vi "Read Latest Frame.vi"(8 "error in (no error)":errorcluster, 9 "Read Timeout (ms)":i32=100, 11 "MJPEG Reader in":refnum<data-value>) -> (0 "error out":errorcluster, 2 "Frame":string, 3 "MJPEG Reader out":refnum<data-value>)   [LabVIEW 2015, in "MJPEG Reader.lvclass"]
uses:
  MJPEG Reader.lvclass
  Get Image State.ctl
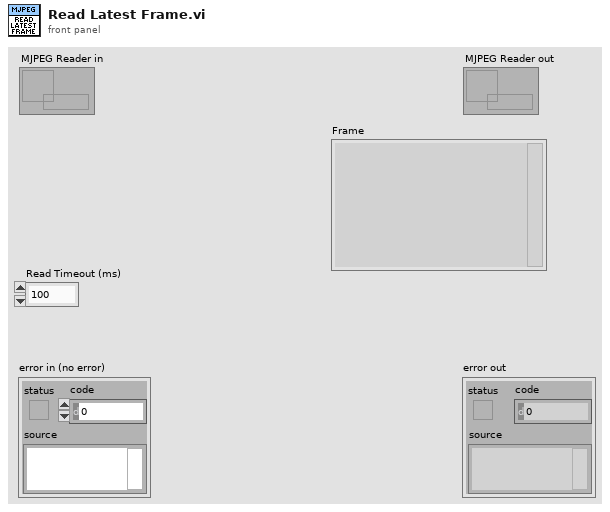
[diagram p1: front panel]
types:
  T1 = typedef "MJPEG Reader.lvclass/Get Image State.ctl" = enum16{"Read First Frame", "Check Most Recent", "Check Image"}
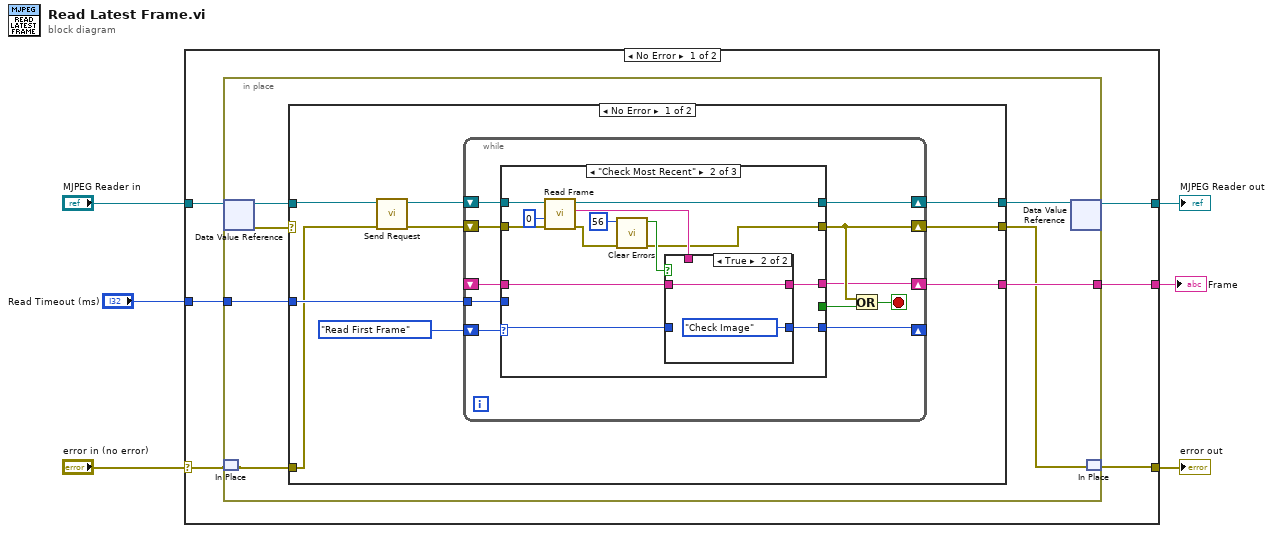
[diagram p0: block diagram]
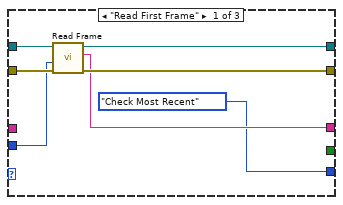
[diagram p2: hidden frame]
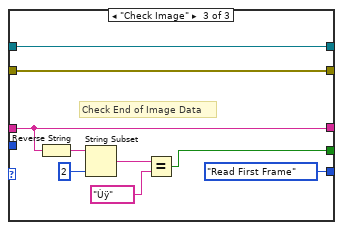
[diagram p4: hidden frame]
diagram:
  n1 = case shown="No Error" "error in (no error)" {
    selector: "error in (no error)" -> [w11 w76]
    tunnel: [w10 w76] -> w5
    tunnel: [w9 w75] -> w3
    tunnel: "MJPEG Reader in" -> [w12 w75]
    tunnel: "Read Timeout (ms)" -> [w8 _]
    tunnel: [w7 _] -> w1
    frame No Error {
      n2 = in-place {
        in-place-border: w8 -> [w15]
        in-place-border: [w14] -> w7
        n3 = in-place-dvr #1(w12) -> (w18:refnum<class "MJPEG Reader.lvclass">, w19:errorcluster)
        n4 = in-place-match #2(w11) -> (w16:errorcluster)
        n5 = case shown="No Error" w19 {
          selector: w19 -> [_ w73]
          tunnel: w18 -> [w23 w74]
          tunnel: w16 -> [w21 _]
          tunnel: [w28 w74] -> w17
          tunnel: w15 -> [w26 _]
          tunnel: [w25 _] -> w14
          tunnel: [w24 w73] -> w13
          frame No Error {
            n6 = call "Send Request.vi"("error in (no error)"=w21, "MJPEG Reader in"=w23) -> ("error out"=w20:errorcluster, "MJPEG Reader out"=w22:refnum<class "MJPEG Reader.lvclass">)  [unwired: 8 in]
            n7 = while {
              shift-right: [w37] -> w28
              shift-left: w22 -> [w39]
              shift-right: [w34] -> w24
              shift-left: w20 -> [w38]
              shift-right: [w30] -> _
              shift-left: Get_Image_State."Read First Frame" ("Get Image State") -> [w36]
              tunnel: w26 -> [w35]
              shift-right: [w32] -> w25
              shift-left: _ -> [w31]
              stop <- w33 stop-if-true
              n8 = case shown="\"Check Most Recent\"" w36 {
                selector: w36 -> [_ w48 _]
                tunnel: w39 -> [w46 w59 w72]
                tunnel: w38 -> [w45 w58 w71]
                tunnel: [w44 w57 w72] -> w37
                tunnel: [w43 w47 w71] -> w34
                tunnel: w35 -> [w42 _ _]
                tunnel: [w41 w51 w70] -> w32
                tunnel: w31 -> [_ w52 w70]
                tunnel: [Get_Image_State."Check Most Recent" ("Get Image State") w50 Get_Image_State."Read First Frame" ("Get Image State")] -> w30
                tunnel: [_ _ w64] -> w29
                frame "Read First Frame" {
                  n9 = call "Read Frame.vi"("error in (no error)"=w45, "Read Timeout (ms)"=w42, "MJPEG Reader in"=w46) -> ("error out"=w43:errorcluster, "Frame"=w41:string, "MJPEG Reader out"=w44:refnum<class "MJPEG Reader.lvclass">)  [unwired: 6 in]
                }
                frame "Check Most Recent" {
                  n10 = call "Read Frame.vi"("error in (no error)"=w58, "Read Timeout (ms)"=0, "MJPEG Reader in"=w59) -> ("error out"=w55:errorcluster, "Frame"=w49:string, "MJPEG Reader out"=w57:refnum<class "MJPEG Reader.lvclass">)  [unwired: 6 in]
                  n11 = call <vilib>:"Clear Errors.vi"("error in (no error)"=w55, "specific error code to clear (0: all)"=56) -> ("error out"=w47:errorcluster, "specific error cleared?"=w53:bool)  [unwired: 4 in]
                  n12 = case shown="True" w53 {
                    tunnel: w52 -> [_ w63]
                    tunnel: [w61 w63] -> w51
                    tunnel: [w60 Get_Image_State."Check Image" ("Get Image State")] -> w50
                    tunnel: w49 -> [w61 _]
                    tunnel: w48 -> [w60 _]
                    frame False {
                    }
                    frame True {
                    }
                  }
                }
                frame "Check Image" {
                  # "Check End of Image Data"
                  n13 = Reverse String(1:w70) -> (0:w69:string)
                  n14 = String Subset(string=w69, length (rest)=2 ("offset (0)")) -> (substring=w67:string)  [unwired: 1 in]
                  n15 = Equal?(x=w67, y="Ùÿ") -> (x = y?=w64:bool)
                }
              }
              n16 = Or(x=w34, y=w29) -> (x .or. y?=w33:bool)
            }
          }
          frame Error {
          }
        }
        n17 = in-place-dvr #1(w17) -> (w9:refnum<data-value>)  [unwired: 1 out]
        n18 = in-place-match #2(w13) -> (w10:errorcluster)
      }
    }
    frame Error {
    }
  }
  "error out" <- w5
  "MJPEG Reader out" <- w3
  "Frame" <- w1
